vi "Read Future.vi"(8 "error in (no error)":errorcluster, 11 "Promise in":refnum<class "Promise.lvclass">) -> (0 "error out":errorcluster, 2 "Future":refnum<class "Future.lvclass">, 3 "Promise out":refnum<class "Promise.lvclass">)   [LabVIEW 2017, in "Promise Future.lvlib" / "Promise.lvclass"]
uses:
  Promise.lvclass
  E:/Promise/Promise Future/Future/Future.lvclass
  Future/Future.lvclass
  Future/Future.lvclass/Future.ctl
  Future/Read Callbacks Queue.vi
  Future/Read Value Queue.vi
  Future/Write Callbacks Queue.vi
  Future/Write Value Queue.vi
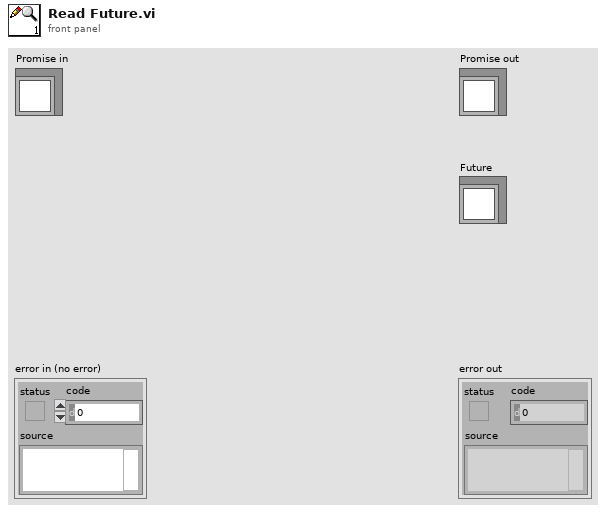
[diagram p1: front panel]
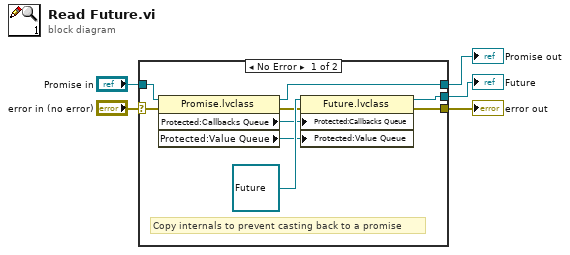
[diagram p0: block diagram]
diagram:
  n1 = case shown="No Error" "error in (no error)" {
    selector: "error in (no error)" -> [w9 w16]
    tunnel: [w8 w16] -> w4
    tunnel: [w6 w15] -> w2
    tunnel: "Promise in" -> [w14 w15]
    tunnel: [w7 _] -> w1
    frame No Error {
      # "Copy internals to prevent casting back to a promise"
      n2 = property class="Promise.lvclass"(reference=w14, error in=w9) -> (reference out=w6:refnum<class "Promise.lvclass">, error out=w10:errorcluster, "Protected:Callbacks Queue"=w12:refnum<queue>, "Protected:Value Queue"=w11:refnum<queue>)
      n3 = property class="Future.lvclass"(reference=refnum<class "Future.lvclass"> refnum ("Future"), error in=w10, "Protected:Callbacks Queue"=w12, "Protected:Value Queue"=w11) -> (reference out=w7:refnum<class "Future.lvclass">, error out=w8:errorcluster)
    }
    frame Error {
    }
  }
  "error out" <- w4
  "Promise out" <- w2
  "Future" <- w1
